vi "test Copy Equal Size.vi"(8 "error in (no error)":errorcluster, 11 "TestCase in":refnum<class "Data Manipulation Tests.lvclass">) -> (0 "error out":errorcluster, 3 "TestCase out":refnum<class "Data Manipulation Tests.lvclass">)   [LabVIEW 2017, in "Pointer Tests.lvlib" / "Data Manipulation Tests.lvclass"]
uses:
  Data Manipulation Tests.lvclass
  Source/Classes/Pointer/Pointer.lvclass/Pointer.ctl
  Source/Classes/Pointer/Public/New/New (4B).vi
  Source/Classes/Pointer/Public/Write/Write (1D I32).vi
  Source/Classes/Pointer/Private/Allocate.vi
  Source/Classes/Pointer/Public/Write (No Check)/Write (No Check 1D I32).vi
  Source/Classes/Pointer/Protected/Parameter Checking/Check Null Pointer.vi
  Source/Classes/Pointer/Protected/Parameter Checking/Check Subset (Power of 2).vi
  Source/Classes/Pointer/API/Accessors/Get Size.vi
  Source/Classes/Pointer/API/Copy Pointer Data.vi
  Source/Classes/Pointer/Public/Compare Size.vi
  Source/Classes/Pointer/API/Read Pointer Data.vi
  Source/Classes/Pointer/Public/Read/Read (1D U8).vi
  Source/Classes/Pointer/Private/Deallocate.vi
  Source/Classes/Pointer/API/Accessors/Set Address.vi
  Source/Classes/Pointer/API/Accessors/Set Size.vi
  Source/Classes/Pointer/Private/Set Internal.vi
  Source/Classes/Pointer/API/Accessors/Get Address.vi
  Source/Classes/Pointer/Protected/Errors.vi
  Source/Classes/Pointer/Protected/Error VIs/Null Pointer.vi
  Source/Classes/Pointer/Protected/Error VIs/Out of Bounds.vi
  Source/Classes/Pointer/Private/Count to Size.vi
  Source/Classes/Pointer/Public/Copy (No Check).vi
  Source/Classes/Pointer/Protected/Parameter Checking/Check Subset.vi
  Source/Classes/Pointer/Protected/Error VIs/Size Mismatch.vi
  Source/Classes/Pointer/Public/Read (No Check)/Read (No Check 1D U8).vi
  Source/Classes/Pointer/Protected/Get Internal.vi
  Source/Classes/Pointer/Protected/Error VIs/Zone.vi
  Source/Classes/Pointer/Protected/Error Building/Create Error.vi
  Source/VIs/Write String into Source.vi
  Source/Classes/Pointer/Protected/Error Building/Write Pointer Size.vi
  Source/VIs/Write Number into Source.vi
  Source/VIs/VIs for Poly/Write U64 into Source.vi
  Source/Constants/Constants.vi
  Source/Constants/Library Name.vi
  Source/Classes/Pointer/Protected/Error Building/Get Error Info.vi
  Source/VIs/Create Error Cluster.vi
  Source/VIs/VIs for Poly/Create Error Cluster (256B).vi
  Source/VIs/Set Error Status.vi
  Source/VIs/Set Error Code.vi
  Source/VIs/Set Error Source.vi
  Source/Classes/Pointer/Pointer.lvclass
  <vilib>/addons/_JKI Toolkits/VI Tester/TestCase.llb/TestCase.lvclass
  C:/Program Files (x86)/National Instruments/LabVIEW 2017/vi.lib/addons/_JKI Toolkits/VI Tester/TestCase.llb/TestCase.lvclass
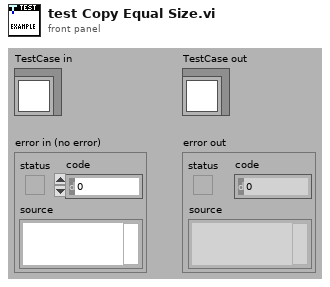
[diagram p1: front panel]
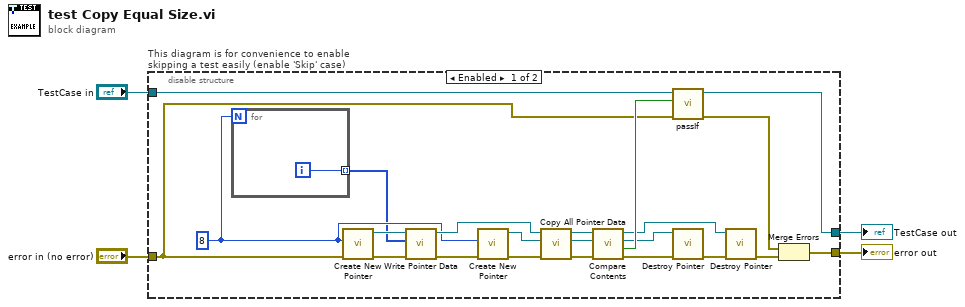
[diagram p0: block diagram]
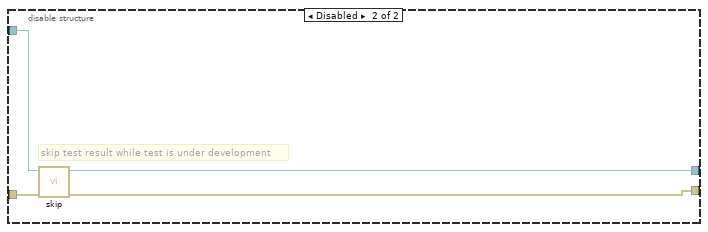
[diagram p2: hidden frame]
diagram:
  n1 = disable-structure "This diagram is for convenience to enable skipping a test easily (enable 'Skip' case)" shown="Enabled" {
    disable-tunnel: "TestCase in" -> [w18 w31]
    disable-tunnel: [w17 w29] -> w1
    disable-tunnel: [w12 w30] -> w3
    disable-tunnel: "error in (no error)" -> [w7 w28]
    frame Enabled {
      w24 = u64 8 ("count (1)")
      n2 = for {
        N: w24 -> [_]
        tunnel: [w27] -> w23 mode=indexing
        i -> [w27]
      }
      n3 = call-poly "Create New Pointer.vi"("error in (no error)"=w7, "count (1)"=w24) -> ("error out"=w15:errorcluster, "Pointer"=w26:refnum<class "Pointer.lvclass">)  [unwired: 8 in]
      n4 = call-poly "Write Pointer Data.vi"("error in (no error)"=w15, "buffer in"=w23, "Pointer in"=w26) -> ("error out"=w14:errorcluster, "Pointer out"=w25:refnum<class "Pointer.lvclass">)  [unwired: 5 in, 2 out]
      n5 = call-poly "Create New Pointer.vi"("error in (no error)"=w14, "count (1)"=w24) -> ("error out"=w13:errorcluster, "Pointer"=w22:refnum<class "Pointer.lvclass">)  [unwired: 8 in]
      n6 = call "Copy All Pointer Data.vi"("error in (no error)"=w13, "dst Pointer in"=w22, "src Pointer in"=w25) -> ("error out"=w10:errorcluster, "dst Pointer out"=w20:refnum<class "Pointer.lvclass">, "src Pointer out"=w21:refnum<class "Pointer.lvclass">)  [unwired: 6 in]
      n7 = call "Compare Contents.vi"("error in (no error)"=w10, "Pointer b in"=w20, "Pointer a in"=w21) -> ("error out"=w11:errorcluster, "equal contents?"=w16:bool, "Pointer b out"=w8:refnum<class "Pointer.lvclass">, "Pointer a out"=w5:refnum<class "Pointer.lvclass">)  [unwired: 5 in]
      n8 = call-dynamic "passIf.vi"("error in (no error)"=w7, "pass"=w16, "TestCase in"=w18) -> ("error out"=w19:errorcluster, "TestCase out"=w17:refnum<class "Data Manipulation Tests.lvclass">)  [unwired: 7 in]
      n9 = call "Destroy Pointer.vi"("error in (no error)"=w11, "Pointer in"=w8) -> ("error out"=w9:errorcluster)  [unwired: 8 in, 1 out]
      n10 = call "Destroy Pointer.vi"("error in (no error)"=w9, "Pointer in"=w5) -> ("error out"=w6:errorcluster)  [unwired: 8 in, 1 out]
      n11 = Merge Errors(w19, w6) -> (w12:errorcluster)
    }
    frame Disabled {
      # "skip test result while test is under development"
      n12 = call <vilib>:"skip.vi"("error in (no error)"=w28, "TestCase in"=w31) -> ("error out"=w30:errorcluster, "TestCase out"=w29:refnum<class "Data Manipulation Tests.lvclass">)  [unwired: 8 in]
    }
  }
  "error out" <- w3
  "TestCase out" <- w1
